vi "Galil DMC Command Generator.vi"(1 "B Deceleration 2":string="20000", 2 "B Acceleration 2":string="10000", 5 "Steer":dbl step=1000.0, 7 "Drive":dbl, 9 "Drive Voltage Decimal Precision":i16) -> (3 "Command String":string, 8 "Maximum Drive Voltage":dbl)   [LabVIEW 2011]
panel:
  out "B Acceleration":string
  out "B Deceleration":string
  out "string":string="PAB="
  out "string 2":string="PAB="
  out "string 3":string="PAB="
  in  "PAC":string="1000"
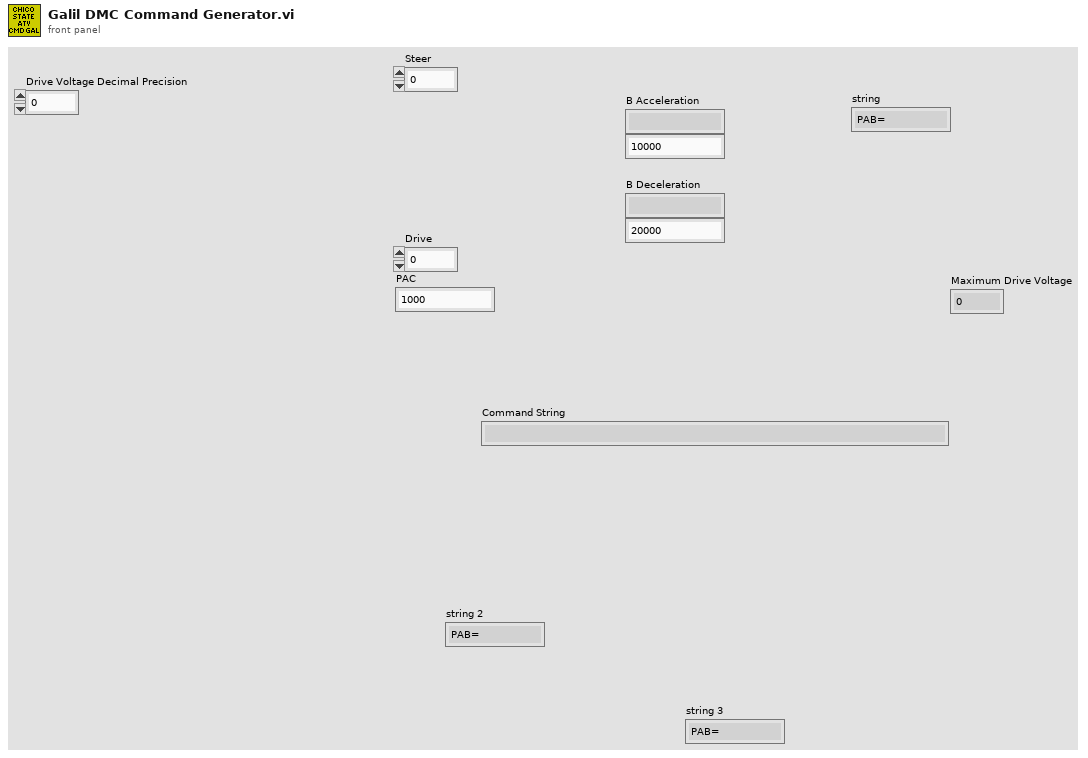
[diagram p1: front panel]
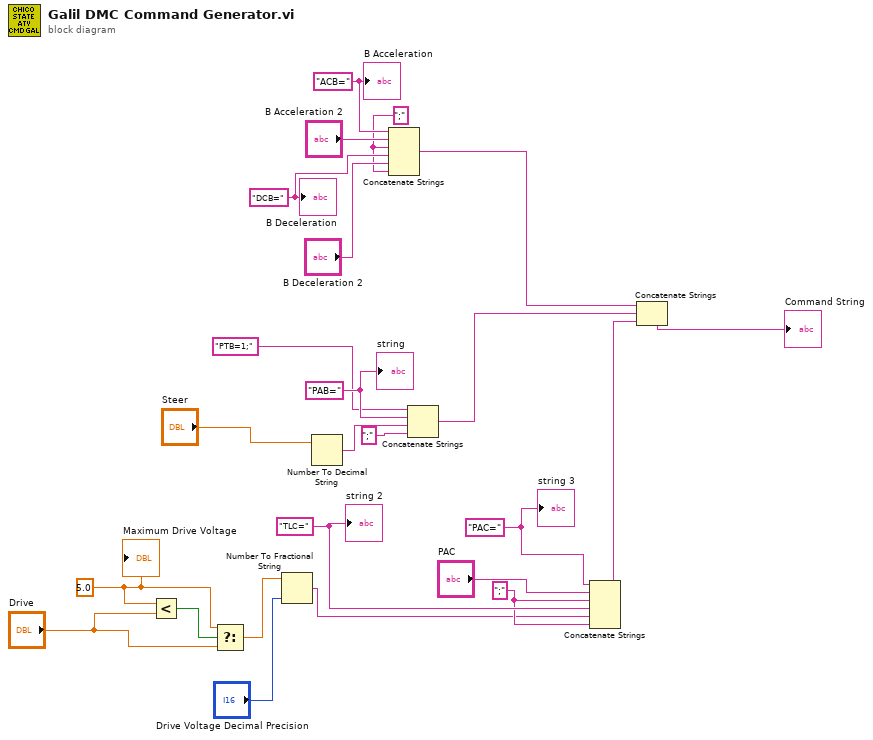
[diagram p0: block diagram]
diagram:
  w4 = ";" ("string")
  w9 = "PAC=" ("string")
  w10 = "TLC=" ("string")
  w12 = 5.0 ("x")
  w17 = "PAB=" ("string")
  w22 = "DCB=" ("string")
  w20 = ";" ("string")
  w23 = "ACB=" ("string")
  n1 = Less?(x=w12, y="Drive") -> (x < y?=w13:bool)
  n2 = Select(t=w12, s=w13, f="Drive") -> (s? t:f=w3:dbl)
  n3 = Number To Fractional String(number=w3, precision (6)="Drive Voltage Decimal Precision") -> (F-format string=w2:string)  [unwired: 2 in]
  n4 = Number To Decimal String(number="Steer") -> (decimal integer string=w16:string)  [unwired: 1 in]
  n5 = Concatenate Strings(w23, "B Acceleration 2", w20, w22, "B Deceleration 2", w20) -> (w19:string)
  n6 = Concatenate Strings("PTB=1;" ("string"), w17, w16, ";" ("string")) -> (w7:string)
  n7 = Concatenate Strings(w9, "PAC", w4, w10, w2, w4) -> (w6:string)
  n8 = Concatenate Strings(w19, w7, w6) -> (→"Command String":string)
  "B Acceleration" <- w23
  "B Deceleration" <- w22
  "string" <- w17
  "Maximum Drive Voltage" <- w12
  "string 2" <- w10
  "string 3" <- w9
